vi "GetLookup table path.vi"() -> (3 "device table path":path)   [LabVIEW 2020]
panel:
  out "Application:Directory Path":path
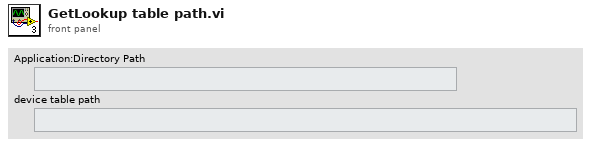
[diagram p1: front panel]
types:
  T1 = enum32{"invalid app kind", "Development System", "Run Time System", "Student Edition", "Embedded LabVIEW", "Evaluation", "Custom"}
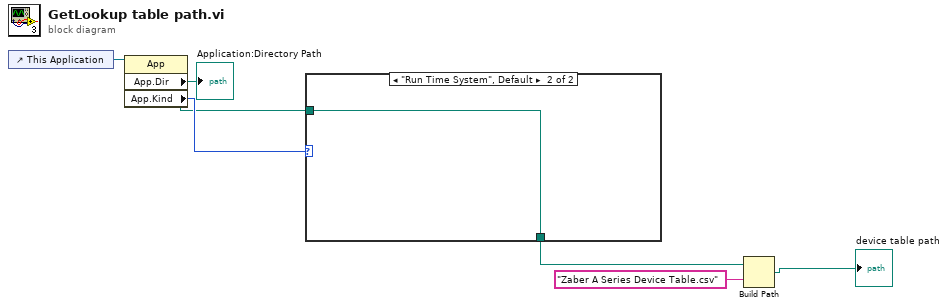
[diagram p0: block diagram]
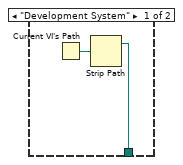
[diagram p2: hidden frame]
diagram:
  n1 = control-ref of="This Application"() -> (w6:refnum<vi>)
  n2 = property class="App"(reference=w6) -> ("App.Dir"=w4:path, "App.Kind"=w5:T1)  [unwired: 1 in, 2 out]
  "Application:Directory Path" <- w4
  n3 = case shown="\"Run Time System\", Default" w5 {
    tunnel: w4 -> [_ w9]
    tunnel: [w7 w9] -> w2
    frame "Development System" {
      n4 = Current VI's Path() -> (path=w8:path)
      n5 = Strip Path(path=w8) -> (stripped path=w7:path)  [unwired: 1 out]
    }
    frame "Run Time System", Default {
    }
  }
  n6 = Build Path(base path=w2, name or relative path="Zaber A Series Device Table.csv") -> (appended path=→"device table path":path)
